vi "From Modbus To Veristand.vi"(7 "Parameters":T1={"Interface Data"={"Name"="", "Unit ID"=0, "Refresh Rate"=0, "Write Rate"=0, "Write Mode"=enum."Value Change", "Interface Type"=enum."TCP Master", "TCP Settings"={"Address"="", "Port"=0, "Timeout"=0}, "Serial Settings"={"VISA resource name"="", "baud rate"=0, "parity (even)"=0, "flow control (none)"=0, "serial type"=enum."RTU", "Wire Mode"=-1}}, "Modbus Input Groups"=[], "Modbus Output Groups"=[], "error in (no error)"={"status"=FALSE, "code"=0, "source"=""}, "Modbus Input Engine Group Names"=[], "Modbus Output Engine Group Names"=[]} {"Modbus Output Groups"."Channel Data"."Mapping"."VS Reference" format="%.0x"; "Modbus Input Groups"."Channel Data"."Mapping"."VS Reference" format="%.0x"; "Interface Data"."Serial Settings"."Wire Mode" items=["Unknown"=-1, "RS485/Wire4"=0, "RS485/Wire2-EchoDTR"=1, "RS485/Wire2-CtrlDTR"=2, "RS485/Wire2-Auto"=3, "RS232/DTE"=128, "RS232/DCE"=129, "RS232/AUTO"=130]; "Interface Data"."Serial Settings"."parity (even)" items=["None", "Odd", "Even", "Mark", "Space"]; "Interface Data"."Serial Settings"."flow control (none)" items=["None", "XON/XOFF", "RTS/CTS", "XON/XOFF & RTS/CTS", "DTR/DSR", "XON/XOFF & DTR/DSR"]}, 8 "error in (no error)":errorcluster, 10 "Process in":refnum<class "Process.lvclass">, 11 "Modbus API.lvlibp:Modbus Master":refnum<class "Modbus Master.lvclass">=refnum) -> ()   [LabVIEW 2021, in "Modbus Master Engine.lvlib"]
uses:
  Modbus Master Engine.lvlib
  <vilib>/NI/NIVS Inline Async API/_VS Inline Async API/Process/Process.lvclass
  Shared/Device Info.ctl
  Shared/Write Mode.ctl
  Shared/Controls/Interface Type.ctl
  Shared/Controls/Data Model/TCP Settings.ctl
  Shared/Controls/Data Model/Serial Settings.ctl
  Bulk Data Access.ctl
  System Explorer/SubVIs/Modbus Type.ctl
  Shared/Controls/Data Model/Channel.ctl
  <vilib>/NI VeriStand/Custom Device API/Custom Device Channel Type.ctl
  Shared/Controls/Data Model/Mapping.ctl
  Shared/Controls/Data Model/DataType.ctl
  <vilib>/NI VeriStand/Custom Device API/Custom Device Item Ref.ctl
  Modbus API.lvlibp/API/Master/Modbus Master.lvclass
  <vilib>/NI/NIVS Inline Async API/_VS Inline Async API/Process/Process.lvclass/Process.ctl
  <vilib>/NI/NIVS Inline Async API/_Data Access Engine/Access Type Classes/Write/Write.lvclass/Write.ctl
  <vilib>/NI/NIVS Inline Async API/_Data Access Engine/Data Access Engine/Methods/Write.Data.vi
  <vilib>/NI/NIVS Inline Async API/_VS Inline Async API/Process/Data Member Access/Read Data Access.vi
  <vilib>/NI/NIVS Inline Async API/_VS Inline Async API/Error Handling Process/SubVIs/Error.ConvertArray.vi
  <vilib>/NI/NIVS Inline Async API/_Data Access Engine/Access Type Classes/Write/Write.ProcessData.vi
  <vilib>/NI/NIVS Inline Async API/_Data Access Engine/Access Type Classes/Write/Write.Buffer.vi
  <vilib>/NI/NIVS Inline Async API/_Data Access Engine/Access Type Classes/Write/Write.Commit.vi
  <vilib>/NI/NIVS Inline Async API/_Data Access Engine/Data Access Engine/Methods/Write.Lookup.vi
  <vilib>/NI/NIVS Inline Async API/_Data Access Engine/Data Access Engine/Data Access Engine.lvclass
  <vilib>/NI/NIVS Inline Async API/_Data Access Engine/Access Type Classes/Write/Write.lvclass
  Shared/Modbus Master Shared.lvlib
  <vilib>/NI VeriStand/Custom Device API/Custom Device API.lvlib
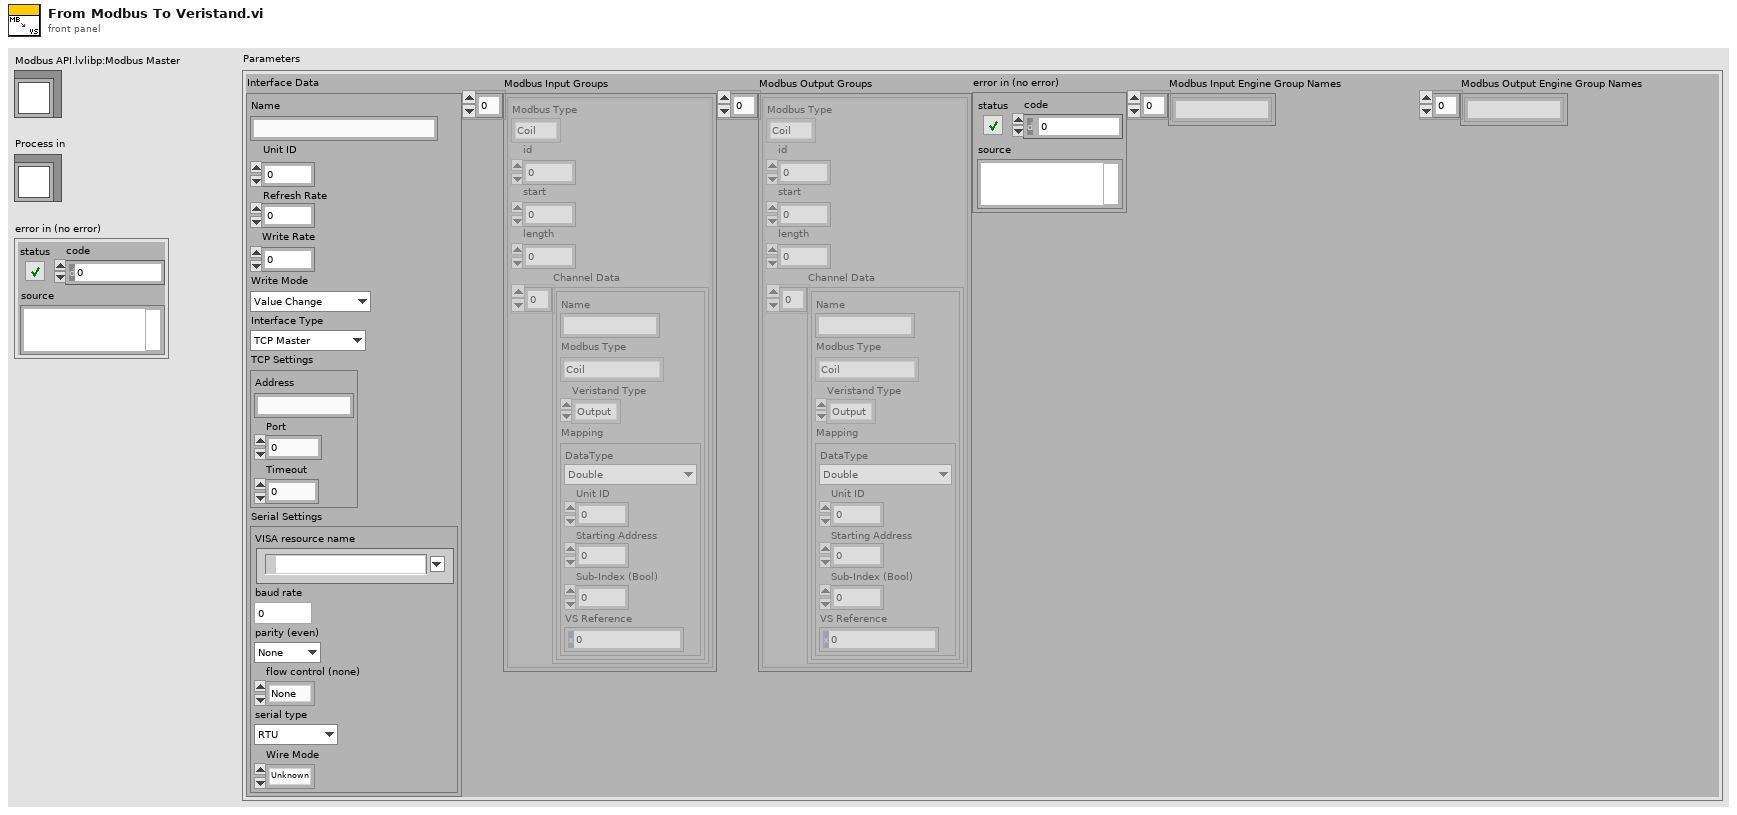
[diagram p1: front panel]
types:
  T1 = typedef "Modbus Master Shared.lvlib/Device Info.ctl" = cluster{"Interface Data":cluster{"Name":string, "Unit ID":u8, "Refresh Rate":i32, "Write Rate":i32, "Write Mode":T2, "Interface Type":T3, "TCP Settings":T4, "Serial Settings":T5}, "Modbus Input Groups":T6[], "Modbus Output Groups":T6[], "error in (no error)":errorcluster, "Modbus Input Engine Group Names":string[], "Modbus Output Engine Group Names":string[]}
  T2 = typedef "Modbus Master Shared.lvlib/Write Mode.ctl" = enum16{"Value Change", "Interval"}
  T3 = typedef "Modbus Master Shared.lvlib/Interface Type.ctl" = enum16{"TCP Master", "Serial Master", "TCP Slave", "Serial Slave"}
  T4 = typedef "Modbus Master Shared.lvlib/TCP Settings.ctl" = cluster{"Address":string, "Port":u16, "Timeout":i32}
  T5 = typedef "Modbus Master Shared.lvlib/Serial Settings.ctl" = cluster{"VISA resource name":refnum<visa-resource-name>, "baud rate":u32, "parity (even)":u16, "flow control (none)":u16, "serial type":enum16{"RTU", "ASCII"}, "Wire Mode":i16}
  T6 = typedef "Modbus Master Shared.lvlib/Bulk Data Access.ctl" = cluster{"Modbus Type":T7, "id":u8, "start":u16, "length":u16, "Channel Data":T8[]}
  T7 = typedef "Modbus Master Shared.lvlib/Modbus Type.ctl" = enum16{"Coil", "Discrete Input", "Holding Register", "Input Register"}
  T8 = typedef "Modbus Master Shared.lvlib/Channel.ctl" = cluster{"Name":string, "Modbus Type":T7, "Veristand Type":T9, "Mapping":T10}
  T9 = typedef "Custom Device API.lvlib/Custom Device Channel Type.ctl" = enum16{"Input", "Output"}
  T10 = typedef "Modbus Master Shared.lvlib/Mapping.ctl" = cluster{"DataType":T11, "Unit ID":u8, "Starting Address":u16, "Sub-Index (Bool)":u16, "VS Reference":T12}
  T11 = typedef "Modbus Master Shared.lvlib/DataType.ctl" = enum16{"Double", "Single", "I64", "I32", "I16", "I8", "U64", "U32", "U16", "U8", "Boolean"}
  T12 = typedef "Custom Device API.lvlib/Custom Device Item Ref.ctl" = u64
  T13 = typedef "Data Access Engine.lvlib/Data Access Engine.lvclass/Write.DVR.ctl" = refnum<data-value>
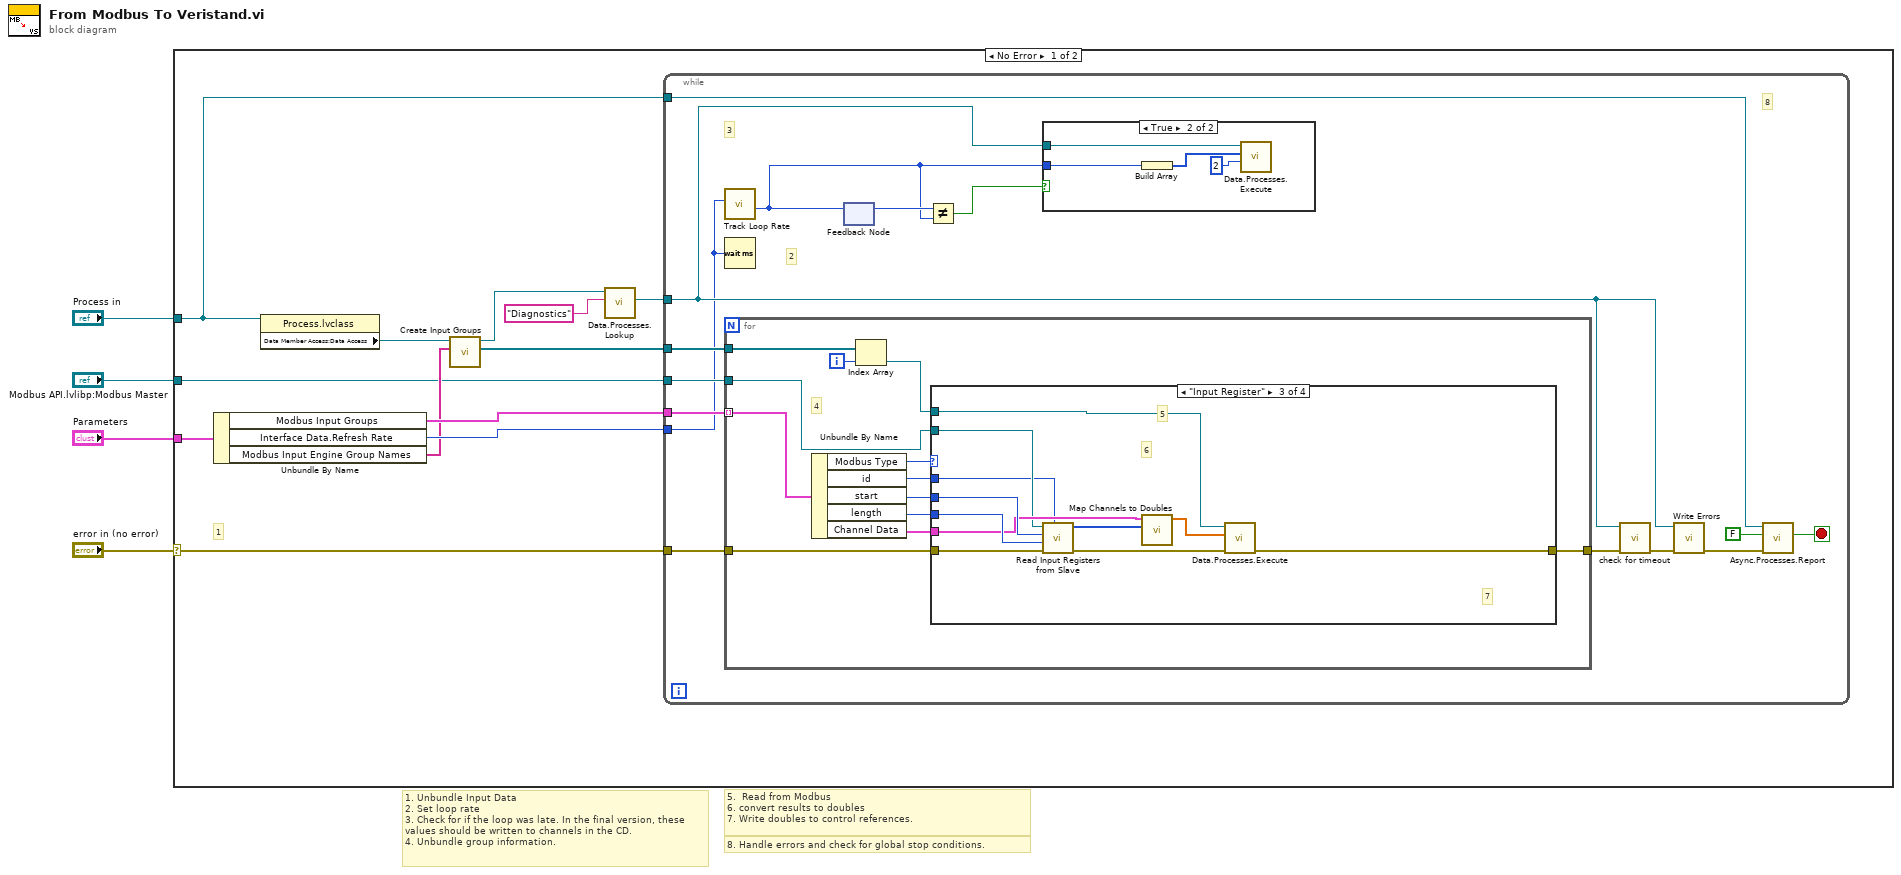
[diagram p0: block diagram]
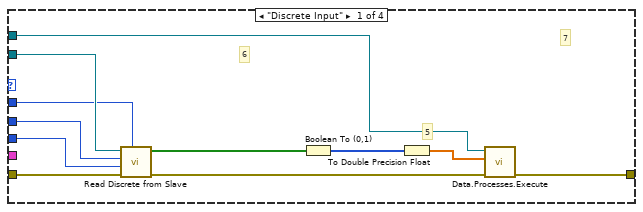
[diagram p3: hidden frame]
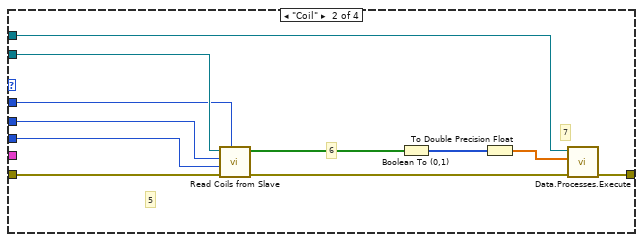
[diagram p4: hidden frame]
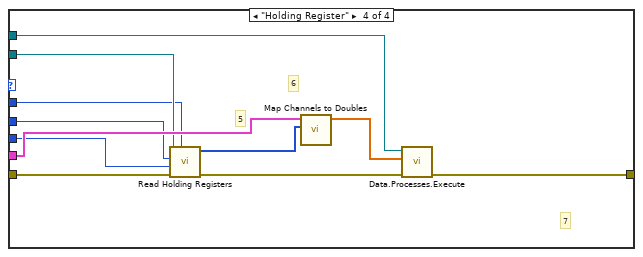
[diagram p5: hidden frame]
diagram:
  # "1. Unbundle Input Data\n2. Set loop rate\n3. Check for if the loop was late. In the final version, these\nvalues should be written to channels in the CD.\n4. Unbundle group information."
  # "5.  Read from Modbus\n6. convert results to doubles\n7. Write doubles to control references."
  # "8. Handle errors and check for global stop conditions."
  n1 = case shown="No Error" "error in (no error)" {
    selector: "error in (no error)" -> [w13 _]
    tunnel: "Parameters" -> [w14 _]
    tunnel: "Process in" -> [w12 _]
    tunnel: "Modbus API.lvlibp:Modbus Master" -> [w5 _]
    frame No Error {
      # "1"
      n2 = Unbundle By Name(w14) -> ("Modbus Input Groups"=w15:T6[], "Interface Data.Refresh Rate"=w16:i32, "Modbus Input Engine Group Names"=w10:string[])
      n3 = property class="Process.lvclass"(reference=w12) -> ("Data Member Access:Data Access"=w11:refnum<class "Data Access Engine.lvclass">)  [unwired: 1 in, 2 out]
      n4 = call "Create Input Groups.vi"("Output Engine Group Names"=w10, "Data Access Engine in"=w11) -> ("Array"=w9:T13[], "Data Access Engine out"=w7:refnum<class "Data Access Engine.lvclass">)  [unwired: 7 in, 1 out]
      n5 = call-poly <vilib>:"Data.Processes.Lookup.vi"("Name"="Diagnostics", "Data Access API in"=w7) -> ("Ref"=w6:T13)  [unwired: 6 in, 3 out]
      n6 = while {
        tunnel: w13 -> [w19]
        tunnel: w12 -> [w31]
        tunnel: w5 -> [w18]
        tunnel: w15 -> [w30]
        tunnel: w9 -> [w29]
        tunnel: w16 -> [w17]
        tunnel: w6 -> [w22]
        stop <- w28 stop-if-true
        # "8"
        # "3"
        # "2"
        n7 = call "Track Loop Rate.vi"("Refresh Rate"=w17) -> ("Late Count"=w24:i32)  [unwired: 8 in, 2 out]
        n8 = Wait (ms)(milliseconds to wait=w17) -> ()  [unwired: 1 out]
        n9 = for {
          tunnel: w30 -> [w47] mode=indexing
          tunnel: w29 -> [w42]
          tunnel: w18 -> [w45]
          tunnel: w19 -> [w37]
          tunnel: [w38] -> w21
          i -> [w40]
          # "4"
          n10 = Unbundle By Name(w47) -> ("Modbus Type"=w46:T7, "id"=w36:u8, "start"=w44:u16, "length"=w43:u16, "Channel Data"=w39:T8[])
          n11 = Index Array(array=w42, index=w40) -> (element=w41:T13)
          n12 = case shown="\"Input Register\"" w46 {
            tunnel: w45 -> [w50 w61 w72 w83]
            tunnel: w44 -> [w54 w63 w79 w82]
            tunnel: w43 -> [w58 w62 w78 w86]
            tunnel: w37 -> [w49 w60 w71 w84]
            tunnel: [w56 w69 w80 w91] -> w38
            tunnel: w41 -> [w53 w68 w77 w90]
            tunnel: w39 -> [_ _ w75 w89]
            tunnel: w36 -> [w48 w59 w70 w81]
            frame "Discrete Input" {
              # "7"
              # "6"
              # "5"
              n13 = call "Read Discrete from Slave.vi"("Unit ID"=w48, "error in (no error)"=w49, "length"=w58, "start"=w54, "Modbus Master in"=w50) -> ("error out"=w57:errorcluster, "discrete inputs"=w55:bool[])  [unwired: 5 in]
              n14 = Boolean To (0,1)(Boolean=w55) -> (0, 1=w51:i16[])
              n15 = To Double Precision Float(number=w51) -> (double precision float=w52:dbl[])
              n16 = call-poly <vilib>:"Data.Processes.Execute.vi"("error in (no error)"=w57, "Values"=w52, "Ref"=w53) -> ("error out"=w56:errorcluster)  [unwired: 8 in]
            }
            frame "Coil" {
              # "7"
              # "6"
              # "5"
              n17 = call "Read Coils from Slave.vi"("Unit ID"=w59, "error in (no error)"=w60, "length"=w62, "start"=w63, "Modbus Master in"=w61) -> ("error out"=w65:errorcluster, "coils"=w64:bool[])  [unwired: 5 in]
              n18 = Boolean To (0,1)(Boolean=w64) -> (0, 1=w66:i16[])
              n19 = To Double Precision Float(number=w66) -> (double precision float=w67:dbl[])
              n20 = call-poly <vilib>:"Data.Processes.Execute.vi"("error in (no error)"=w65, "Values"=w67, "Ref"=w68) -> ("error out"=w69:errorcluster)  [unwired: 8 in]
            }
            frame "Input Register" {
              # "7"
              # "6"
              # "5"
              n21 = call "Read Input Registers from Slave.vi"("Unit ID"=w70, "error in (no error)"=w71, "length"=w78, "start"=w79, "Modbus Master in"=w72) -> ("error out"=w76:errorcluster, "register values"=w74:u16[])  [unwired: 5 in]
              n22 = call "Map Channels to Doubles.vi"("register values"=w74, "Channel Data"=w75) -> ("Array"=w73:dbl[])  [unwired: 9 in]
              n23 = call-poly <vilib>:"Data.Processes.Execute.vi"("error in (no error)"=w76, "Values"=w73, "Ref"=w77) -> ("error out"=w80:errorcluster)  [unwired: 8 in]
            }
            frame "Holding Register" {
              # "7"
              # "6"
              # "5"
              n24 = call "Read Holding Registers.vi"("Unit ID"=w81, "error in (no error)"=w84, "length"=w86, "start"=w82, "Modbus Master in"=w83) -> ("error out"=w85:errorcluster, "register values"=w87:u16[])  [unwired: 5 in]
              n25 = call "Map Channels to Doubles.vi"("register values"=w87, "Channel Data"=w89) -> ("Array"=w88:dbl[])  [unwired: 9 in]
              n26 = call-poly <vilib>:"Data.Processes.Execute.vi"("error in (no error)"=w85, "Values"=w88, "Ref"=w90) -> ("error out"=w91:errorcluster)  [unwired: 8 in]
            }
          }
        }
        n27 = feedback-in #1(w24) -> ()
        n28 = feedback #1() -> (w26:i32)  [unwired: 1 in]
        n29 = Not Equal?(x=w26, y=w24) -> (x != y?=w25:bool)
        n30 = case shown="True" w25 {
          tunnel: w22 -> [_ w35]
          tunnel: w24 -> [_ w33]
          frame False {
          }
          frame True {
            n31 = Build Array(w33) -> (w32:i32[])
            n32 = call-poly <vilib>:"Data.Processes.Execute.vi"("Offset"=2, "Values"=w32, "Ref"=w35) -> ()  [unwired: 8 in, 1 out]
          }
        }
        n33 = call "check for timeout.vi"("error in (no error)"=w21, "Data Value Reference in"=w22) -> ("error out"=w20:errorcluster)  [unwired: 9 in]
        n34 = call "Write Errors.vi"("error in (no error)"=w20, "Data Value Reference in"=w22) -> ("error out"=w23:errorcluster)  [unwired: 9 in]
        n35 = call <vilib>:"Async.Processes.Report.vi"("Error"=w23, "Stop Async on Error?"=FALSE ("Stop on Error?"), "Process in"=w31) -> ("Stop"=w28:bool)  [unwired: 7 in, 1 out]
      }
    }
    frame Error {
    }
  }
